vi "ConstructorString.vi"(6 "error in":errorcluster, 9 "ForLoop in":refnum<class "ForLoop.lvclass">) -> (0 "error out":errorcluster, 3 "ForLoop out":refnum<class "ForLoop.lvclass">, 4 "constructor":string)   [LabVIEW 2014, in "Raspberry Pi Compatible Compiler for LabVIEW.lvlib" / "ForLoop.lvclass"]
uses:
  ForLoop.lvclass
  ForLoop.lvclass/ForLoop.ctl
  Python/Parsing/ListTypesTD.ctl
  Python/Parsing/Python Functions.lvlib
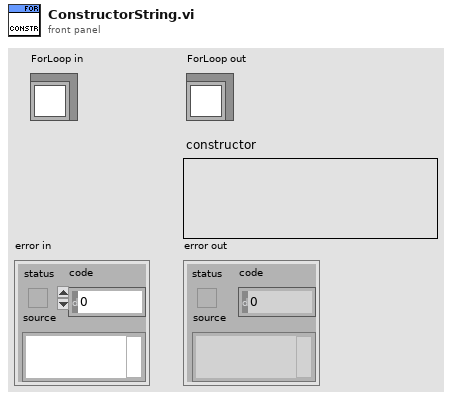
[diagram p1: front panel]
types:
  T1 = typedef "Raspberry Pi Compatible Compiler for LabVIEW.lvlib/Python Functions.lvlib/ListTypesTD.ctl" = enum16{"list", "tuple", "parameter list", "output list", "return values"}
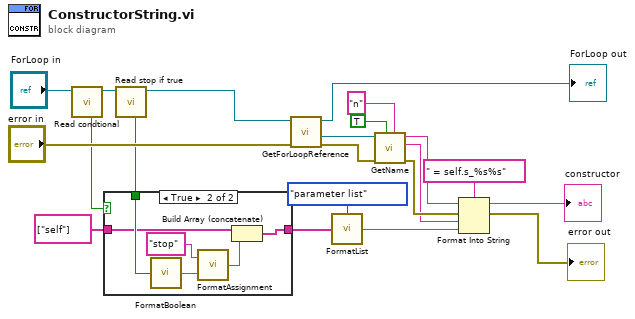
[diagram p0: block diagram]
diagram:
  n1 = call "Read condtional.vi"("ForLoop in"="ForLoop in") -> ("ForLoop out"=w6:refnum<class "ForLoop.lvclass">, "condtional"=w4:bool)  [unwired: 7 in]
  n2 = call "Read stop if true.vi"("ForLoop in"=w6) -> ("ForLoop out"=w5:refnum<class "ForLoop.lvclass">, "stop if true"=w2:bool)  [unwired: 7 in]
  n3 = case shown="True" w4 {
    tunnel: [w22 w23] -> w3
    tunnel: w2 -> [_ w26]
    tunnel: string[] ["self"] ("values") -> [w22 w25]
    frame False {
    }
    frame True {
      n4 = call "FormatBoolean.vi"("value"=w26) -> ("python object"=w28:string)
      n5 = call "FormatAssignment.vi"("value"=w28, "name"="stop") -> ("python assignment"=w24:string)
      n6 = Build Array (concatenate)(w25, w24) -> (w23:string[])
    }
  }
  n7 = call "GetForLoopReference.vi"("error in"="error in", "ForLoop in"=w5) -> ("error out"=w13:errorcluster, "reference out"=w14:refnum<vi>, "ForLoop out"=→"ForLoop out":refnum<class "ForLoop.lvclass">)  [unwired: 7 in]
  n8 = call "FormatList.vi"("values"=w3, "type"=ListTypesTD."parameter list") -> ("python object"=w19:string)
  n9 = call "GetName.vi"("base name"="n", "add self"=TRUE, "error in"=w13, "GObj Refnum"=w14) -> ("error out"=w12:errorcluster, "UID"=w8:string, "name"=w9:string)  [unwired: 5 in]
  n10 = Format Into String(format string=" = self.s_%s%s", initial string=w9, error in=w12, w8, w19) -> (resulting string=→"constructor":string, error out=→"error out":errorcluster)
